vi "_CSMObj-Is Group Alive.vi"(8 "error in (no error)":errorcluster, 11 "CSMQ In":T1) -> (0 "error out":errorcluster, 2 "Group Alive?":bool, 3 "CSMQ Out":T1)   [LabVIEW 2017, in "Communicable State Machine.lvlib"]
uses:
  Communicable State Machine.lvlib
  _CSMObj.ctl
  _CSMObj-Info.ctl
  Typedef/_CSM_MODE.ctl
  _CSMObj-Refs.ctl
  _CSMObj-Data.ctl
  Priority Queue/Priority Queue.ctl
  Typedef/_Cross CSM State Data.ctl
  Typedef/_CSM_MSG_TYPE.ctl
  Typedef/_Cross CSM State Response.ctl
  Typedef/_CSM_Response Source Message.ctl
  Priority Queue/def-Data(LowPRI-Q).ctl
  _CSMObj-ModeData.ctl
  Typedef/_CSM Status Change Event Data.ctl
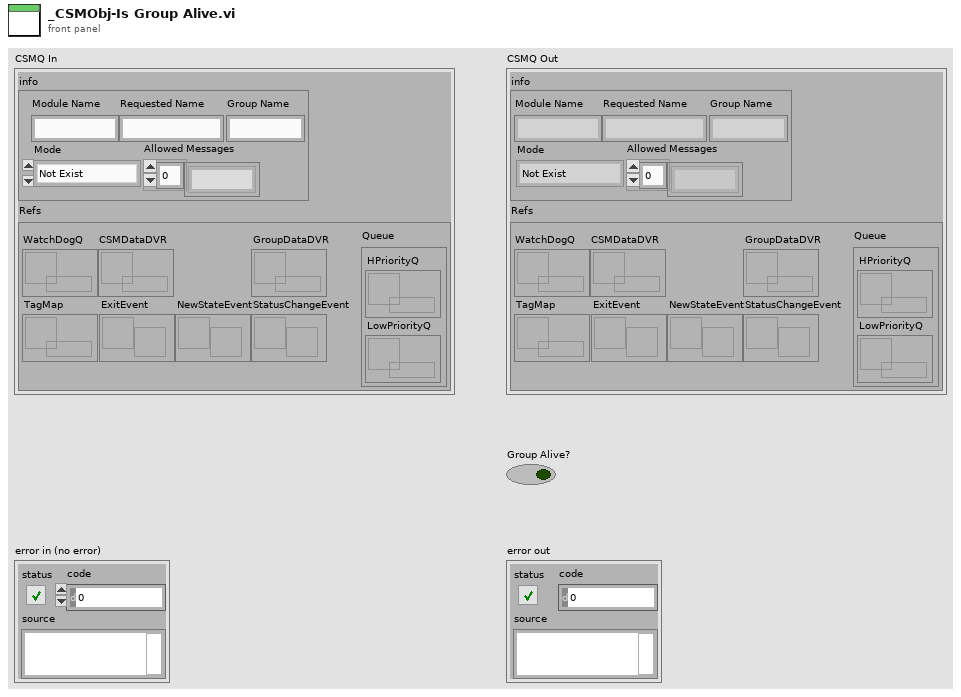
[diagram p1: front panel]
types:
  T1 = typedef "Communicable State Machine.lvlib/_CSMObj.ctl" = cluster{"info":T2, "Refs":T4}
  T2 = typedef "Communicable State Machine.lvlib/_CSMObj-Info.ctl" = cluster{"Module Name":string, "Requested Name":string, "Group Name":string, "Mode":T3, "Allowed Messages":string[]}
  T3 = typedef "Communicable State Machine.lvlib/_CSM_MODE.ctl" = enum16{"Not Exist", "Stand Alone", "CSM", "Worker", "Worker Agent", "Chain Node", "Chain"}
  T4 = typedef "Communicable State Machine.lvlib/_CSMObj-Refs.ctl" = cluster{"WatchDogQ":refnum<queue>, "CSMDataDVR":refnum<data-value>, "Queue":T5, "GroupDataDVR":refnum<data-value>, "TagMap":refnum<data-value>, "ExitEvent":refnum<user-event>, "NewStateEvent":refnum<user-event>, "StatusChangeEvent":refnum<user-event>}
  T5 = typedef "Communicable State Machine.lvlib/Priority Queue.ctl" = cluster{"HPriorityQ":refnum<queue>, "LowPriorityQ":refnum<queue>}
  T6 = typedef "Communicable State Machine.lvlib/_CSMObj-ModeData.ctl" = cluster{"CSMDataDVR":refnum<data-value>[], "Messages of Chain Nodes":cluster{"Module Name":string, "Allowed Messages":string[]}[], "Chain Message Mapping Map":variant}
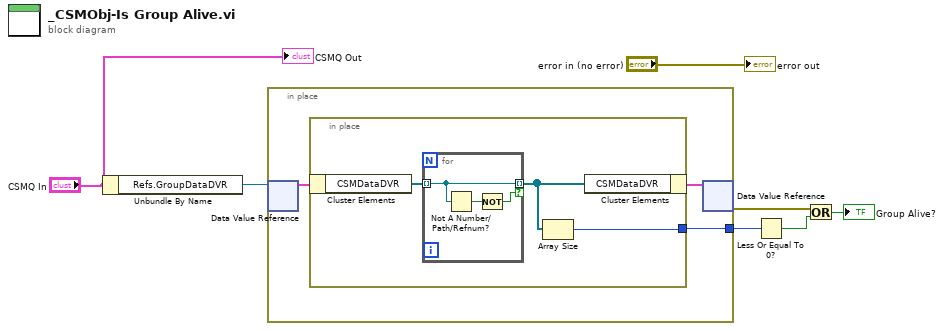
[diagram p0: block diagram]
diagram:
  n1 = Unbundle By Name("CSMQ In") -> ("Refs.GroupDataDVR"=w7:refnum<data-value>)
  n2 = in-place "In Place Element Structure" {
    in-place-border: [w8] -> w3
    n3 = in-place-dvr #1(w7) -> (w10:T6)  [unwired: 1 out]
    n4 = in-place {
      in-place-border: [w11] -> w8
      n5 = in-place-cluster #2(w10) -> ("CSMDataDVR"=w13:refnum<data-value>[])
      n6 = for {
        tunnel: [w16] -> w12 mode=indexing if=w14
        tunnel: w13 -> [w16] mode=indexing
        n7 = Not A Number/Path/Refnum?(number/path/refnum=w16) -> (NaN/Path/Refnum?=w15:bool)
        n8 = Not(x=w15) -> (.not. x?=w14:bool)
      }
      n9 = Array Size(array=w12) -> (size(s)=w11:i32)
      n10 = in-place-cluster #2("CSMDataDVR"=w12) -> (w9:T6)
    }
    n11 = in-place-dvr #1(w9) -> (w6:errorcluster)  [unwired: 1 out]
  }
  n12 = Less Or Equal To 0?(x=w3) -> (x <= 0?=w4:bool)
  n13 = Or(x=w6, y=w4) -> (x .or. y?=→"Group Alive?":bool)
  "error out" <- "error in (no error)"
  "CSMQ Out" <- "CSMQ In"
